vi "Srednia.vi"() -> ()   [LabVIEW 2017, in "GUI.lvlib"]
uses:
  Libraries/GUI/GUI.lvlib
  Libraries/Akwizycja/Data Enum.ctl
  <vilib>/Delacor/Delacor QMH/Libraries/Message Queue_class/Delacor_lib_QMH_Enqueue Message (Single).vi
  <vilib>/Delacor/Delacor QMH/Libraries/Message Queue_class/Delacor_lib_QMH_Message Queue.lvclass
panel:
  out "Średnia 24H":T1
  out "Średnia 16H":T2
  out "Średnia 8H":T3
  out "Średnia 4H":T4
  out "Średnia 1H":T5
  out "avg flows":T6
  out "avg temps":T6
  in  "Avg fuel":T6
  in  "output cluster":T6
  in  "Automatyczne przełączanie":bool
  in  "Czas przełączania":dbl=15.0 min=15.0 max=600.0 step=1.0
  in  "Stop":bool
  in  "Podgląd":T7
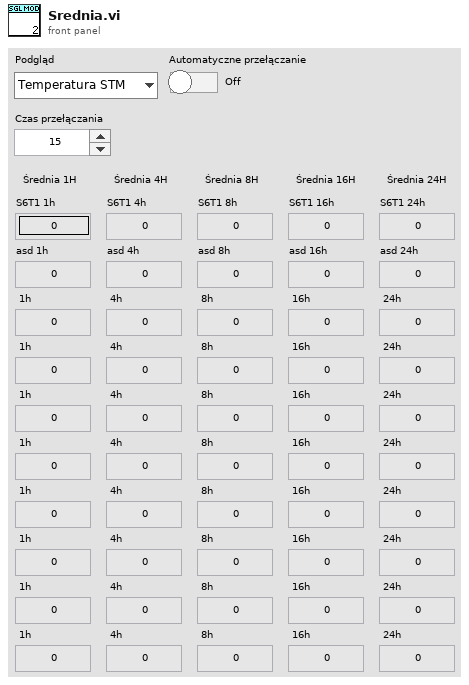
[diagram p1: front panel]
types:
  T1 = cluster{"Zmienna 51":dbl, "Zmienna 52":dbl, "Zmienna 53":dbl, "Zmienna 54":dbl, "Zmienna 55":dbl, "Zmienna 56":dbl, "Zmienna 57":dbl, "Zmienna 58":dbl, "Zmienna 59":dbl, "Zmienna 60":dbl}
  T2 = cluster{"Zmienna 41":dbl, "Zmienna 42":dbl, "Zmienna 43":dbl, "Zmienna 44":dbl, "Zmienna 45":dbl, "Zmienna 46":dbl, "Zmienna 47":dbl, "Zmienna 48":dbl, "Zmienna 49":dbl, "Zmienna 50":dbl}
  T3 = cluster{"Zmienna 31":dbl, "Zmienna 32":dbl, "Zmienna 33":dbl, "Zmienna 34":dbl, "Zmienna 35":dbl, "Zmienna 36":dbl, "Zmienna 37":dbl, "Zmienna 38":dbl, "Zmienna 39":dbl, "Zmienna 40":dbl}
  T4 = cluster{"Zmienna 21":dbl, "Zmienna 22":dbl, "Zmienna 23":dbl, "Zmienna 24":dbl, "Zmienna 25":dbl, "Zmienna 26":dbl, "Zmienna 27":dbl, "Zmienna 28":dbl, "Zmienna 29":dbl, "Zmienna 30":dbl}
  T5 = cluster{"Zmienna 11":dbl, "Zmienna 12":dbl, "Zmienna 13":dbl, "Zmienna 14":dbl, "Zmienna 15":dbl, "Zmienna 16":dbl, "Zmienna 17":dbl, "Zmienna 18":dbl, "Zmienna 19":dbl, "Zmienna 20":dbl}
  T6 = cluster{"24h avg":dbl[][], "16h avg":dbl[][], "8h avg":dbl[][], "4h avg":dbl[][], "1h avg":dbl[][]}
  T7 = typedef "Podgląd średnie typedef.ctl" = enum16{"Temperatura STM", "Temperatura S2", "Temperatura S3", "Temperatura S4", "Temperatura S5", "Temperatura S6", "Przepływ S2", "Przepływ S3", "Przepływ S4", "Przepływ S5", "Przepływ S6"}
  T8 = typedef "Data Enum.ctl" = enum16{"get_data", "get_data_switch"}
  T9 = cluster{"Controls[]":refnum<vi>[], "Controls[]":refnum<vi>[], "Controls[]":refnum<vi>[], "Controls[]":refnum<vi>[], "Controls[]":refnum<vi>[]}
  T10 = cluster{"24h avg[0]":dbl, "24h avg[1]":dbl, "24h avg[2]":dbl, "24h avg[3]":dbl, "24h avg[4]":dbl, "24h avg[5]":dbl, "24h avg[6]":dbl, "24h avg[7]":dbl, "24h avg[8]":dbl, "24h avg[9]":dbl}
  T11 = cluster{"16h avg[0]":dbl, "16h avg[1]":dbl, "16h avg[2]":dbl, "16h avg[3]":dbl, "16h avg[4]":dbl, "16h avg[5]":dbl, "16h avg[6]":dbl, "16h avg[7]":dbl, "16h avg[8]":dbl, "16h avg[9]":dbl}
  T12 = cluster{"8h avg[0]":dbl, "8h avg[1]":dbl, "8h avg[2]":dbl, "8h avg[3]":dbl, "8h avg[4]":dbl, "8h avg[5]":dbl, "8h avg[6]":dbl, "8h avg[7]":dbl, "8h avg[8]":dbl, "8h avg[9]":dbl}
  T13 = cluster{"4h avg[0]":dbl, "4h avg[1]":dbl, "4h avg[2]":dbl, "4h avg[3]":dbl, "4h avg[4]":dbl, "4h avg[5]":dbl, "4h avg[6]":dbl, "4h avg[7]":dbl, "4h avg[8]":dbl, "4h avg[9]":dbl}
  T14 = cluster{"1h avg[0]":dbl, "1h avg[1]":dbl, "1h avg[2]":dbl, "1h avg[3]":dbl, "1h avg[4]":dbl, "1h avg[5]":dbl, "1h avg[6]":dbl, "1h avg[7]":dbl, "1h avg[8]":dbl, "1h avg[9]":dbl}
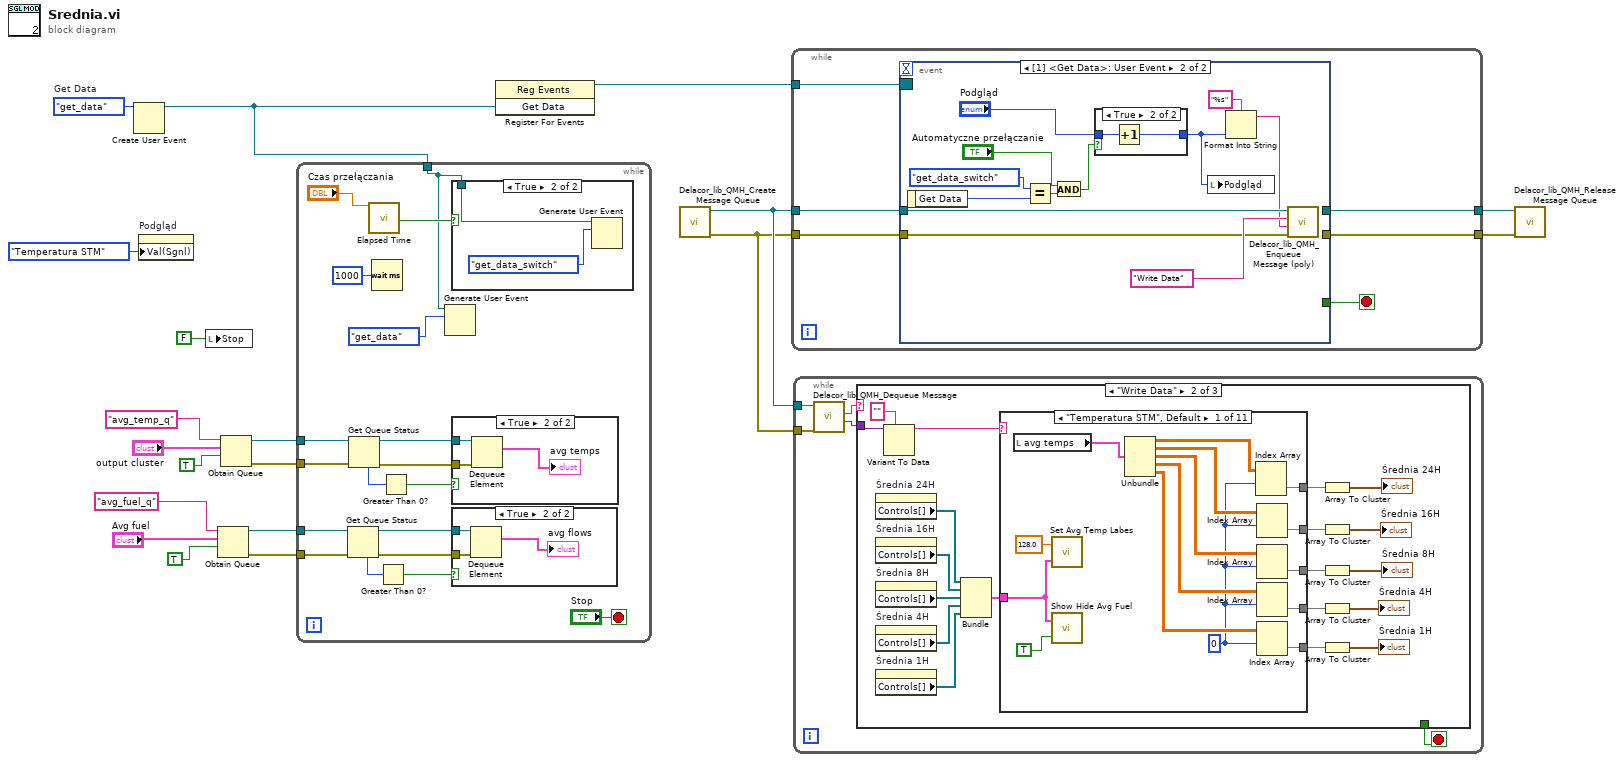
[diagram p0: block diagram]
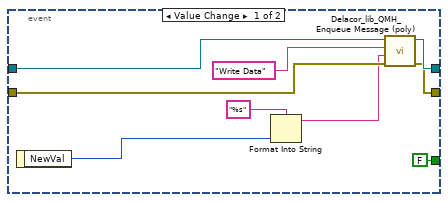
[diagram p5: hidden frame]
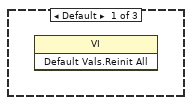
[diagram p7: hidden frame]
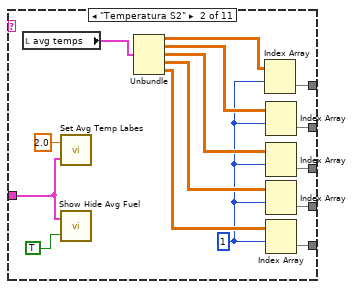
[diagram p8: hidden frame]
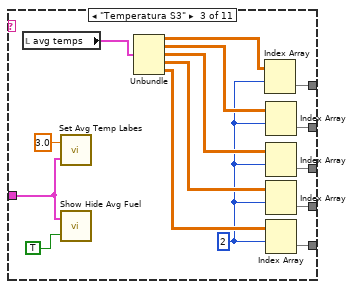
[diagram p9: hidden frame]
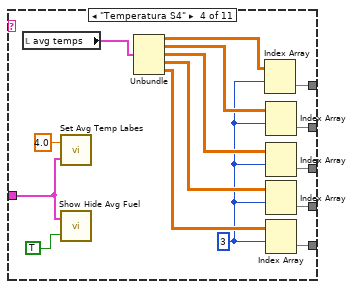
[diagram p10: hidden frame]
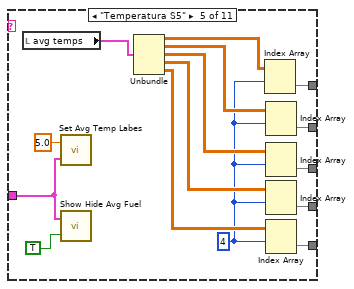
[diagram p11: hidden frame]
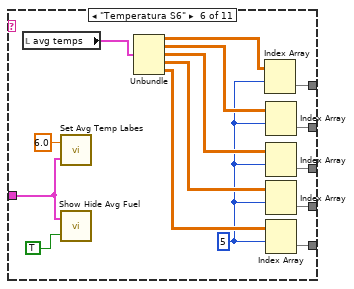
[diagram p12: hidden frame]
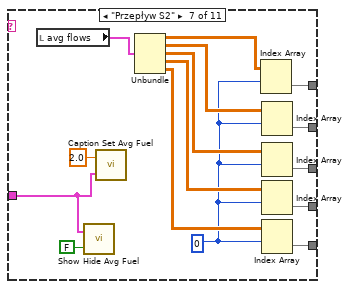
[diagram p13: hidden frame]
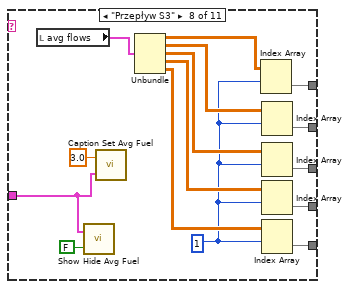
[diagram p14: hidden frame]
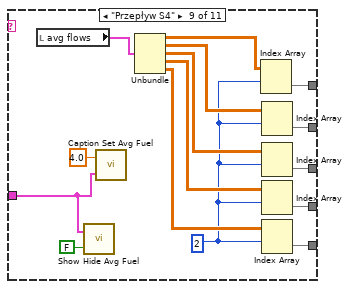
[diagram p15: hidden frame]
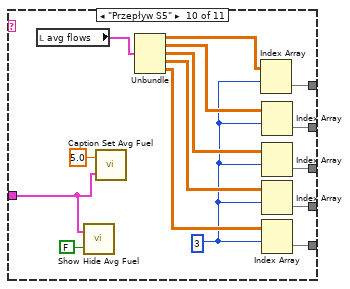
[diagram p16: hidden frame]
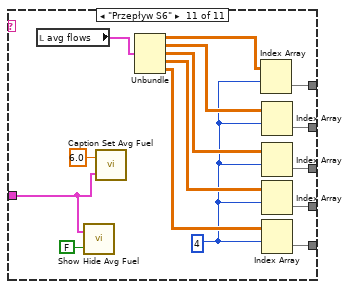
[diagram p17: hidden frame]
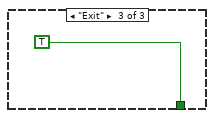
[diagram p18: hidden frame]
diagram:
  w11 = Data_Enum."get_data"  # Get Data
  n1 = Create User Event(user event datatype=w11) -> (user event=w6:refnum<user-event>)  [unwired: 1 in, 1 out]
  n2 = property on="Podgląd" class="Enum (strict)"("Val(Sgnl)"=Podgląd_średnie_typedef."Temperatura STM" ("Value (Signaling)")) -> ()  [unwired: 2 in, 2 out]
  n3 = local write "Stop"(FALSE) -> ()
  n4 = Obtain Queue(name (unnamed)="avg_fuel_q", element data type="Avg fuel", create if not found? (T)=TRUE) -> (queue out=w13:refnum<queue>, error out=w12:errorcluster)  [unwired: 2 in, 1 out]
  n5 = Obtain Queue(name (unnamed)="avg_temp_q", element data type="output cluster", create if not found? (T)=TRUE) -> (queue out=w16:refnum<queue>, error out=w15:errorcluster)  [unwired: 2 in, 1 out]
  n6 = while {
    tunnel: w16 -> [w33]
    tunnel: w15 -> [w32]
    tunnel: w13 -> [w26]
    tunnel: w12 -> [w27]
    tunnel: w6 -> [w21]
    stop <- "Stop" stop-if-true
    n7 = Get Queue Status(queue=w26, error in (no error)=w27) -> (queue out=w22:refnum<queue>, error out=w23:errorcluster, # elements in queue=w25:i32)  [unwired: 1 in, 5 out]
    n8 = Get Queue Status(queue=w33, error in (no error)=w32) -> (queue out=w29:refnum<queue>, error out=w30:errorcluster, # elements in queue=w31:i32)  [unwired: 1 in, 5 out]
    n9 = call "Elapsed Time"("Time Target (s)"="Czas przełączania") -> ("Time has Elapsed"=w36:bool)  [unwired: 11 in, 7 out]
    n10 = Wait (ms)(milliseconds to wait=u32 1000) -> ()  [unwired: 1 out]
    n11 = Greater Than 0?(x=w25) -> (x > 0?=w24:bool)
    n12 = Greater Than 0?(x=w31) -> (x > 0?=w28:bool)
    n13 = Generate User Event(user event=w21, event data cluster=Data_Enum."get_data" ("event data")) -> ()  [unwired: 2 in, 2 out]
    n14 = case shown="True" w36 {
      tunnel: w21 -> [_ w45]
      frame False {
      }
      frame True {
        n15 = Generate User Event(user event=w45, event data cluster=Data_Enum."get_data_switch") -> ()  [unwired: 2 in, 2 out]
      }
    }
    n16 = case shown="True" w28 {
      tunnel: w30 -> [_ w43]
      tunnel: w29 -> [_ w42]
      frame False {
      }
      frame True {
        n17 = Dequeue Element(queue=w42, error in (no error)=w43) -> (element=→"avg temps":T6)  [unwired: 1 in, 3 out]
      }
    }
    n18 = case shown="True" w24 {
      tunnel: w22 -> [_ w40]
      tunnel: w23 -> [_ w39]
      frame False {
      }
      frame True {
        n19 = Dequeue Element(queue=w40, error in (no error)=w39) -> (element=→"avg flows":T6)  [unwired: 1 in, 3 out]
      }
    }
  }
  n20 = register-events(w6) -> (reference out=w19:refnum<event-registration>)  [unwired: 2 in, 1 out]
  n21 = call <vilib>:"Delacor_lib_QMH_Create Message Queue.vi"() -> ("error out"=w9:errorcluster, "Message Queue"=w10:refnum<class "Delacor_lib_QMH_Message Queue.lvclass">)  [unwired: 10 in]
  n22 = while {
    tunnel: w10 -> [w51]
    tunnel: w9 -> [w50]
    tunnel: [w49] -> w8
    tunnel: [w48] -> w7
    tunnel: w19 -> [w46]
    stop <- w47 stop-if-true
    n23 = event shown="[1] <Get Data>: User Event" {
      selector: w46 -> [_ _]
      dyn-events: _ -> [_ _]
      timeout: _ -> [_ _]
      tunnel: w51 -> [w59 w70]
      tunnel: w50 -> [w58 w71]
      tunnel: [w57 _] -> w49
      tunnel: [w56 _] -> w48
      tunnel: [FALSE _] -> w47
      event Value Change {
        n24 = event-data() -> ("NewVal"=w54:T7)  [unwired: 1 in]
        n25 = Format Into String(format string="%s", w54) -> (resulting string=w52:string)  [unwired: 2 in, 1 out]
        n26 = call-poly <vilib>:"Delacor_lib_QMH_Enqueue Message (poly).vi"("error in (no error)"=w58, "Message Data"=w52, "Message"="Write Data", "Message Queue in"=w59) -> ("error out"=w56:errorcluster, "Message Queue out"=w57:refnum<class "Delacor_lib_QMH_Message Queue.lvclass">)  [unwired: 6 in]
      }
      event User Event {
        n27 = event-data() -> ("Get Data"=w65:T8)  [unwired: 1 in]
        n28 = Equal?(x=Data_Enum."get_data_switch", y=w65) -> (x = y?=w63:bool)
        n29 = And(x="Automatyczne przełączanie", y=w63) -> (x .and. y?=w61:bool)
        n30 = case shown="True" w61 {
          tunnel: "Podgląd" -> [w73 w75]
          tunnel: [w73 w74] -> w67
          frame False {
          }
          frame True {
            n31 = Increment(x=w75) -> (x+1=w74:T7)
          }
        }
        n32 = local write "Podgląd"(w67) -> ()
        n33 = Format Into String(format string="%s", w67) -> (resulting string=w69:string)  [unwired: 2 in, 1 out]
        n34 = call-poly <vilib>:"Delacor_lib_QMH_Enqueue Message (poly).vi"("error in (no error)"=w71, "Message Data"=w69, "Message"="Write Data", "Message Queue in"=w70) -> ()  [unwired: 6 in, 2 out]
      }
    }
  }
  n35 = while {
    tunnel: w10 -> [w80]
    tunnel: w9 -> [w79]
    stop <- w76 stop-if-true
    n36 = call-dynamic "Delacor_lib_QMH_Dequeue Message.vi"("error in (no error)"=w79, "Message Queue in"=w80) -> ("Message Data"=w78:variant, "Message"=w77:string)  [unwired: 6 in, 2 out]
    n37 = case shown="\"Write Data\"" w77 {
      tunnel: w78 -> [_ w99 _]
      tunnel: [_ _ TRUE] -> w76
      frame Default {
        n38 = invoke class="VI" method="Default Vals.Reinit All"() -> ()  [unwired: 3 in, 3 out]
      }
      frame "Write Data" {
        n39 = property on="Średnia 24H" class="Clust (strict)"() -> ("Controls[]"=w87:refnum<vi>[])  [unwired: 2 in, 2 out]
        n40 = property on="Średnia 16H" class="Clust (strict)"() -> ("Controls[]"=w86:refnum<vi>[])  [unwired: 2 in, 2 out]
        n41 = property on="Średnia 8H" class="Clust (strict)"() -> ("Controls[]"=w85:refnum<vi>[])  [unwired: 2 in, 2 out]
        n42 = property on="Średnia 4H" class="Clust (strict)"() -> ("Controls[]"=w83:refnum<vi>[])  [unwired: 2 in, 2 out]
        n43 = property on="Średnia 1H" class="Clust (strict)"() -> ("Controls[]"=w84:refnum<vi>[])  [unwired: 2 in, 2 out]
        n44 = Variant To Data(type="", Variant=w99) -> (data=w81:string)  [unwired: 1 in, 1 out]
        n45 = Bundle("Controls[]"=w87, "Controls[]"=w86, "Controls[]"=w85, "Controls[]"=w83, "Controls[]"=w84) -> (w82:T9)  [unwired: 1 in]
        n46 = case shown="\"Temperatura STM\", Default" w81 {
          tunnel: [w114 w129 w144 w159 w174 w189 w204 w219 w234 w249 w264] -> w97
          tunnel: [w113 w128 w143 w158 w173 w188 w203 w218 w233 w248 w263] -> w96
          tunnel: [w112 w127 w142 w157 w172 w187 w202 w217 w232 w247 w262] -> w95
          tunnel: [w111 w126 w141 w156 w171 w186 w201 w216 w231 w246 w261] -> w94
          tunnel: [w110 w125 w140 w155 w170 w185 w200 w215 w230 w245 w260] -> w93
          tunnel: w82 -> [w100 w115 w130 w145 w160 w175 w191 w206 w221 w236 w251]
          frame "Temperatura STM", Default {
            w103 = 0 ("index (row)")
            n47 = local read "avg temps"() -> (w109:T6)
            n48 = call "Set Avg Temp Labes.vi"("Reference Cluster"=w100, "Slave ID"=128.0) -> ()
            n49 = call "Show Hide Avg Fuel.vi"("Bool"=TRUE, "Reference Cluster"=w100) -> ()
            n50 = Unbundle(w109) -> ("24h avg"=w108:dbl[][], "16h avg"=w107:dbl[][], "8h avg"=w106:dbl[][], "4h avg"=w105:dbl[][], "1h avg"=w104:dbl[][])
            n51 = Index Array(array=w108, index (row)=w103) -> (element=w114:dbl[])  [unwired: 1 in]
            n52 = Index Array(array=w107, index (row)=w103) -> (element=w113:dbl[])  [unwired: 1 in]
            n53 = Index Array(array=w106, index (row)=w103) -> (element=w112:dbl[])  [unwired: 1 in]
            n54 = Index Array(array=w105, index (row)=w103) -> (element=w111:dbl[])  [unwired: 1 in]
            n55 = Index Array(array=w104, index (row)=w103) -> (element=w110:dbl[])  [unwired: 1 in]
          }
          frame "Temperatura S2" {
            w118 = 1 ("index (row)")
            n56 = local read "avg temps"() -> (w124:T6)
            n57 = call "Set Avg Temp Labes.vi"("Reference Cluster"=w115, "Slave ID"=2.0) -> ()
            n58 = call "Show Hide Avg Fuel.vi"("Bool"=TRUE, "Reference Cluster"=w115) -> ()
            n59 = Unbundle(w124) -> ("24h avg"=w123:dbl[][], "16h avg"=w122:dbl[][], "8h avg"=w121:dbl[][], "4h avg"=w120:dbl[][], "1h avg"=w119:dbl[][])
            n60 = Index Array(array=w123, index (row)=w118) -> (element=w129:dbl[])  [unwired: 1 in]
            n61 = Index Array(array=w122, index (row)=w118) -> (element=w128:dbl[])  [unwired: 1 in]
            n62 = Index Array(array=w121, index (row)=w118) -> (element=w127:dbl[])  [unwired: 1 in]
            n63 = Index Array(array=w120, index (row)=w118) -> (element=w126:dbl[])  [unwired: 1 in]
            n64 = Index Array(array=w119, index (row)=w118) -> (element=w125:dbl[])  [unwired: 1 in]
          }
          frame "Temperatura S3" {
            w133 = 2 ("index (row)")
            n65 = local read "avg temps"() -> (w139:T6)
            n66 = call "Set Avg Temp Labes.vi"("Reference Cluster"=w130, "Slave ID"=3.0) -> ()
            n67 = call "Show Hide Avg Fuel.vi"("Bool"=TRUE, "Reference Cluster"=w130) -> ()
            n68 = Unbundle(w139) -> ("24h avg"=w138:dbl[][], "16h avg"=w137:dbl[][], "8h avg"=w136:dbl[][], "4h avg"=w135:dbl[][], "1h avg"=w134:dbl[][])
            n69 = Index Array(array=w138, index (row)=w133) -> (element=w144:dbl[])  [unwired: 1 in]
            n70 = Index Array(array=w137, index (row)=w133) -> (element=w143:dbl[])  [unwired: 1 in]
            n71 = Index Array(array=w136, index (row)=w133) -> (element=w142:dbl[])  [unwired: 1 in]
            n72 = Index Array(array=w135, index (row)=w133) -> (element=w141:dbl[])  [unwired: 1 in]
            n73 = Index Array(array=w134, index (row)=w133) -> (element=w140:dbl[])  [unwired: 1 in]
          }
          frame "Temperatura S4" {
            w148 = 3 ("index (row)")
            n74 = local read "avg temps"() -> (w154:T6)
            n75 = call "Set Avg Temp Labes.vi"("Reference Cluster"=w145, "Slave ID"=4.0) -> ()
            n76 = call "Show Hide Avg Fuel.vi"("Bool"=TRUE, "Reference Cluster"=w145) -> ()
            n77 = Unbundle(w154) -> ("24h avg"=w153:dbl[][], "16h avg"=w152:dbl[][], "8h avg"=w151:dbl[][], "4h avg"=w150:dbl[][], "1h avg"=w149:dbl[][])
            n78 = Index Array(array=w153, index (row)=w148) -> (element=w159:dbl[])  [unwired: 1 in]
            n79 = Index Array(array=w152, index (row)=w148) -> (element=w158:dbl[])  [unwired: 1 in]
            n80 = Index Array(array=w151, index (row)=w148) -> (element=w157:dbl[])  [unwired: 1 in]
            n81 = Index Array(array=w150, index (row)=w148) -> (element=w156:dbl[])  [unwired: 1 in]
            n82 = Index Array(array=w149, index (row)=w148) -> (element=w155:dbl[])  [unwired: 1 in]
          }
          frame "Temperatura S5" {
            w163 = 4 ("index (row)")
            n83 = local read "avg temps"() -> (w169:T6)
            n84 = call "Set Avg Temp Labes.vi"("Reference Cluster"=w160, "Slave ID"=5.0) -> ()
            n85 = call "Show Hide Avg Fuel.vi"("Bool"=TRUE, "Reference Cluster"=w160) -> ()
            n86 = Unbundle(w169) -> ("24h avg"=w168:dbl[][], "16h avg"=w167:dbl[][], "8h avg"=w166:dbl[][], "4h avg"=w165:dbl[][], "1h avg"=w164:dbl[][])
            n87 = Index Array(array=w168, index (row)=w163) -> (element=w174:dbl[])  [unwired: 1 in]
            n88 = Index Array(array=w167, index (row)=w163) -> (element=w173:dbl[])  [unwired: 1 in]
            n89 = Index Array(array=w166, index (row)=w163) -> (element=w172:dbl[])  [unwired: 1 in]
            n90 = Index Array(array=w165, index (row)=w163) -> (element=w171:dbl[])  [unwired: 1 in]
            n91 = Index Array(array=w164, index (row)=w163) -> (element=w170:dbl[])  [unwired: 1 in]
          }
          frame "Temperatura S6" {
            w178 = 5 ("index (row)")
            n92 = local read "avg temps"() -> (w184:T6)
            n93 = call "Set Avg Temp Labes.vi"("Reference Cluster"=w175, "Slave ID"=6.0) -> ()
            n94 = call "Show Hide Avg Fuel.vi"("Bool"=TRUE, "Reference Cluster"=w175) -> ()
            n95 = Unbundle(w184) -> ("24h avg"=w183:dbl[][], "16h avg"=w182:dbl[][], "8h avg"=w181:dbl[][], "4h avg"=w180:dbl[][], "1h avg"=w179:dbl[][])
            n96 = Index Array(array=w183, index (row)=w178) -> (element=w189:dbl[])  [unwired: 1 in]
            n97 = Index Array(array=w182, index (row)=w178) -> (element=w188:dbl[])  [unwired: 1 in]
            n98 = Index Array(array=w181, index (row)=w178) -> (element=w187:dbl[])  [unwired: 1 in]
            n99 = Index Array(array=w180, index (row)=w178) -> (element=w186:dbl[])  [unwired: 1 in]
            n100 = Index Array(array=w179, index (row)=w178) -> (element=w185:dbl[])  [unwired: 1 in]
          }
          frame "Przepływ S2" {
            w193 = 0 ("index (row)")
            n101 = local read "avg flows"() -> (w199:T6)
            n102 = call "Show Hide Avg Fuel.vi"("Bool"=FALSE, "Reference Cluster"=w191) -> ()
            n103 = call "Caption Set Avg Fuel.vi"("Reference Cluster"=w191, "Slave ID"=2.0) -> ()
            n104 = Unbundle(w199) -> ("24h avg"=w198:dbl[][], "16h avg"=w197:dbl[][], "8h avg"=w196:dbl[][], "4h avg"=w195:dbl[][], "1h avg"=w194:dbl[][])
            n105 = Index Array(array=w198, index (row)=w193) -> (element=w204:dbl[])  [unwired: 1 in]
            n106 = Index Array(array=w197, index (row)=w193) -> (element=w203:dbl[])  [unwired: 1 in]
            n107 = Index Array(array=w196, index (row)=w193) -> (element=w202:dbl[])  [unwired: 1 in]
            n108 = Index Array(array=w195, index (row)=w193) -> (element=w201:dbl[])  [unwired: 1 in]
            n109 = Index Array(array=w194, index (row)=w193) -> (element=w200:dbl[])  [unwired: 1 in]
          }
          frame "Przepływ S3" {
            w208 = 1 ("index (row)")
            n110 = local read "avg flows"() -> (w214:T6)
            n111 = call "Show Hide Avg Fuel.vi"("Bool"=FALSE, "Reference Cluster"=w206) -> ()
            n112 = call "Caption Set Avg Fuel.vi"("Reference Cluster"=w206, "Slave ID"=3.0) -> ()
            n113 = Unbundle(w214) -> ("24h avg"=w213:dbl[][], "16h avg"=w212:dbl[][], "8h avg"=w211:dbl[][], "4h avg"=w210:dbl[][], "1h avg"=w209:dbl[][])
            n114 = Index Array(array=w213, index (row)=w208) -> (element=w219:dbl[])  [unwired: 1 in]
            n115 = Index Array(array=w212, index (row)=w208) -> (element=w218:dbl[])  [unwired: 1 in]
            n116 = Index Array(array=w211, index (row)=w208) -> (element=w217:dbl[])  [unwired: 1 in]
            n117 = Index Array(array=w210, index (row)=w208) -> (element=w216:dbl[])  [unwired: 1 in]
            n118 = Index Array(array=w209, index (row)=w208) -> (element=w215:dbl[])  [unwired: 1 in]
          }
          frame "Przepływ S4" {
            w223 = 2 ("index (row)")
            n119 = local read "avg flows"() -> (w229:T6)
            n120 = call "Show Hide Avg Fuel.vi"("Bool"=FALSE, "Reference Cluster"=w221) -> ()
            n121 = call "Caption Set Avg Fuel.vi"("Reference Cluster"=w221, "Slave ID"=4.0) -> ()
            n122 = Unbundle(w229) -> ("24h avg"=w228:dbl[][], "16h avg"=w227:dbl[][], "8h avg"=w226:dbl[][], "4h avg"=w225:dbl[][], "1h avg"=w224:dbl[][])
            n123 = Index Array(array=w228, index (row)=w223) -> (element=w234:dbl[])  [unwired: 1 in]
            n124 = Index Array(array=w227, index (row)=w223) -> (element=w233:dbl[])  [unwired: 1 in]
            n125 = Index Array(array=w226, index (row)=w223) -> (element=w232:dbl[])  [unwired: 1 in]
            n126 = Index Array(array=w225, index (row)=w223) -> (element=w231:dbl[])  [unwired: 1 in]
            n127 = Index Array(array=w224, index (row)=w223) -> (element=w230:dbl[])  [unwired: 1 in]
          }
          frame "Przepływ S5" {
            w238 = 3 ("index (row)")
            n128 = local read "avg flows"() -> (w244:T6)
            n129 = call "Show Hide Avg Fuel.vi"("Bool"=FALSE, "Reference Cluster"=w236) -> ()
            n130 = call "Caption Set Avg Fuel.vi"("Reference Cluster"=w236, "Slave ID"=5.0) -> ()
            n131 = Unbundle(w244) -> ("24h avg"=w243:dbl[][], "16h avg"=w242:dbl[][], "8h avg"=w241:dbl[][], "4h avg"=w240:dbl[][], "1h avg"=w239:dbl[][])
            n132 = Index Array(array=w243, index (row)=w238) -> (element=w249:dbl[])  [unwired: 1 in]
            n133 = Index Array(array=w242, index (row)=w238) -> (element=w248:dbl[])  [unwired: 1 in]
            n134 = Index Array(array=w241, index (row)=w238) -> (element=w247:dbl[])  [unwired: 1 in]
            n135 = Index Array(array=w240, index (row)=w238) -> (element=w246:dbl[])  [unwired: 1 in]
            n136 = Index Array(array=w239, index (row)=w238) -> (element=w245:dbl[])  [unwired: 1 in]
          }
          frame "Przepływ S6" {
            w253 = 4 ("index (row)")
            n137 = local read "avg flows"() -> (w259:T6)
            n138 = call "Show Hide Avg Fuel.vi"("Bool"=FALSE, "Reference Cluster"=w251) -> ()
            n139 = call "Caption Set Avg Fuel.vi"("Reference Cluster"=w251, "Slave ID"=6.0) -> ()
            n140 = Unbundle(w259) -> ("24h avg"=w258:dbl[][], "16h avg"=w257:dbl[][], "8h avg"=w256:dbl[][], "4h avg"=w255:dbl[][], "1h avg"=w254:dbl[][])
            n141 = Index Array(array=w258, index (row)=w253) -> (element=w264:dbl[])  [unwired: 1 in]
            n142 = Index Array(array=w257, index (row)=w253) -> (element=w263:dbl[])  [unwired: 1 in]
            n143 = Index Array(array=w256, index (row)=w253) -> (element=w262:dbl[])  [unwired: 1 in]
            n144 = Index Array(array=w255, index (row)=w253) -> (element=w261:dbl[])  [unwired: 1 in]
            n145 = Index Array(array=w254, index (row)=w253) -> (element=w260:dbl[])  [unwired: 1 in]
          }
        }
        n146 = Array To Cluster(array=w97) -> (cluster=→"Średnia 24H":T10)
        n147 = Array To Cluster(array=w96) -> (cluster=→"Średnia 16H":T11)
        n148 = Array To Cluster(array=w95) -> (cluster=→"Średnia 8H":T12)
        n149 = Array To Cluster(array=w94) -> (cluster=→"Średnia 4H":T13)
        n150 = Array To Cluster(array=w93) -> (cluster=→"Średnia 1H":T14)
      }
      frame "Exit" {
      }
    }
  }
  n151 = call-dynamic "Delacor_lib_QMH_Release Message Queue.vi"("error in (no error)"=w7, "Message Queue"=w8) -> ()  [unwired: 9 in, 1 out]
